vi "myRIO v1.0 Config Manager Encoder.vi"(7 "Action":T1, 10 "Encoder Signal Mode":T2, 11 "Encoder Channel":T3) -> (3 "Success?":bool)   [LabVIEW 2021]
uses:
  <vilib>/myRIO/Common/Instrument Driver Framework/myRIO v1.0/Encoder/typedefs/Encoder Channels Enum.ctl
  <vilib>/myRIO/Common/Instrument Driver Framework/myRIO v1.0/Encoder/typedefs/Encoder Signal Mode.ctl
  <vilib>/myRIO/Common/Instrument Driver Framework/myRIO v1.0/Encoder/typedefs/Encoder Config Manager Action Enum.ctl
  <vilib>/myRIO/Common/Instrument Driver Framework/myRIO v1.0/Encoder/typedefs/Encoder Config Cache Data.ctl
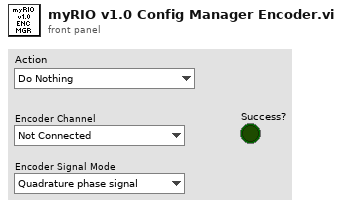
[diagram p1: front panel]
types:
  T1 = typedef "Encoder Config Manager Action Enum.ctl" = enum16{"Do Nothing", "Store", "Clear"}
  T2 = typedef "Encoder Signal Mode.ctl" = enum16{"Quadrature phase signal", "Step and direction signal"}
  T3 = typedef "Encoder Channels Enum.ctl" = enum16{"Not Connected", "C/ENC0", "C/ENC1", "A/ENC", "A/ENC0", "A/ENC1", "A/ENC2", "A/ENC3", "A/ENC4", "A/ENC5", "A/ENC6", "A/ENC7", "A/ENC8", "A/ENC9", "B/ENC", "B/ENC0", "B/ENC1", "B/ENC2", "B/ENC3", "B/ENC4", "B/ENC5", "B/ENC6", "B/ENC7", "B/ENC8", "B/ENC9", "DIO/ENC0", "DIO/ENC1", "DIO/ENC2", "DIO/ENC3", "DIO/ENC4"}
  T4 = typedef "Encoder Config Cache Data.ctl" = cluster{"Set?":bool, "Encoder Signal Mode":T2}
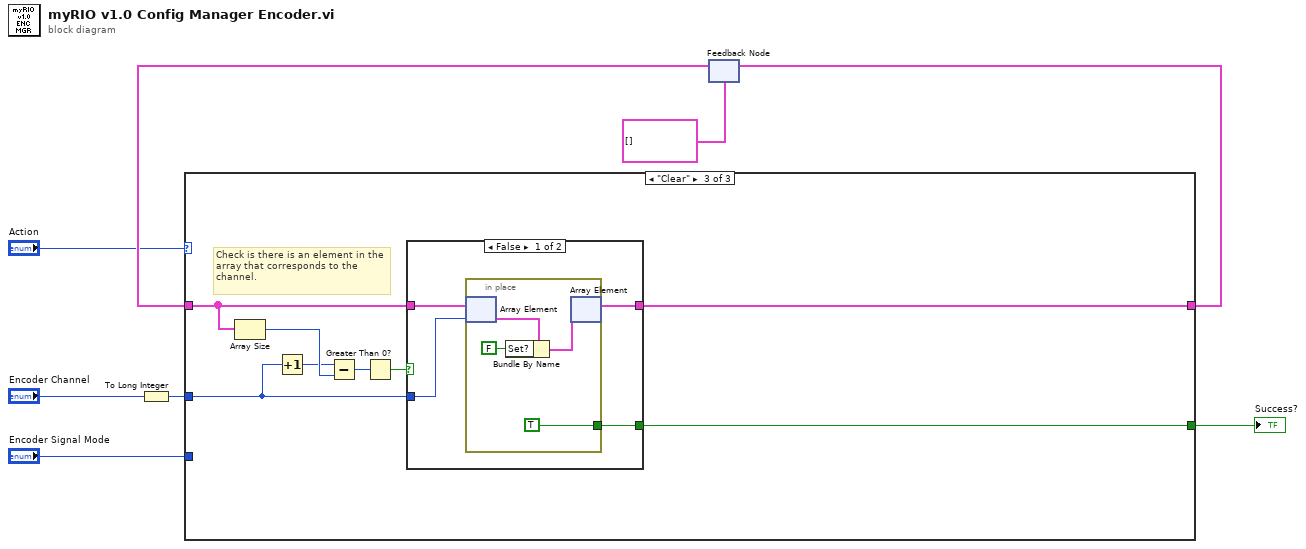
[diagram p0: block diagram]
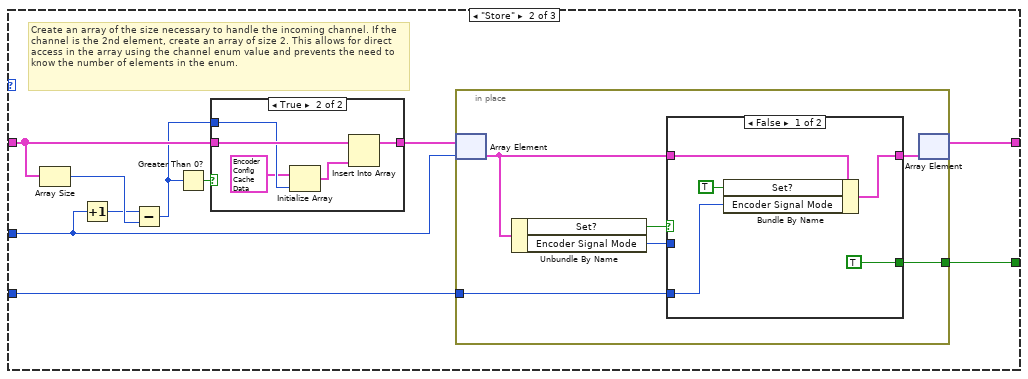
[diagram p3: hidden frame]
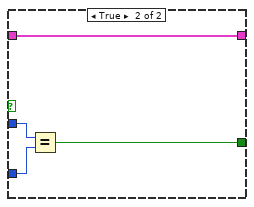
[diagram p5: hidden frame]
diagram:
  n1 = To Long Integer(number="Encoder Channel") -> (32bit integer=w3:i32)
  n2 = feedback #1(T4[] []) -> (w7:T4[])
  n3 = case shown="\"Clear\"" "Action" {
    tunnel: w7 -> [w9 w16 w45]
    tunnel: w3 -> [_ w11 w42]
    tunnel: "Encoder Signal Mode" -> [_ w19 _]
    tunnel: [w9 w18 w44] -> w5
    tunnel: [_ w10 w41] -> w2
    frame "Do Nothing", Default {
    }
    frame "Store" {
      # "Create an array of the size necessary to handle the incoming channel. If the channel is the 2nd element, create an array of size 2. This allows for direct access in the array using the channel enum value and prevents the need to know the number of elements in the enum."
      n4 = Array Size(array=w16) -> (size(s)=w15:i32)
      n5 = Increment(x=w11) -> (x+1=w12:i32)
      n6 = Subtract(x=w12, y=w15) -> (x-y=w14:i32)
      n7 = Greater Than 0?(x=w14) -> (x > 0?=w13:bool)
      n8 = case shown="True" w13 {
        tunnel: [w20 w24] -> w17
        tunnel: w16 -> [w20 w25]
        tunnel: w14 -> [_ w23]
        frame False {
        }
        frame True {
          n9 = Initialize Array(T4 {"Set?"=FALSE, "Encoder Signal Mode"=enum."Quadrature phase signal"}, w23) -> (w22:T4[])
          n10 = Insert Into Array(array=w25, new element=w22) -> (w24:T4[])  [unwired: 1 in]
        }
      }
      n11 = in-place {
        in-place-border: w19 -> [w29]
        in-place-border: [w26] -> w10
        n12 = in-place-array #2(w17, w11) -> (w28:T4)
        n13 = Unbundle By Name(w28) -> ("Set?"=w31:bool, "Encoder Signal Mode"=w30:T2)
        n14 = case shown="False" w31 {
          tunnel: w30 -> [_ w40]
          tunnel: w29 -> [w34 w39]
          tunnel: w28 -> [w36 w38]
          tunnel: [w35 w38] -> w27
          tunnel: [TRUE ("Set?") w37] -> w26
          frame False {
            n15 = Bundle By Name(cluster=w36, "Set?"=TRUE, "Encoder Signal Mode"=w34) -> (w35:T4)
          }
          frame True {
            n16 = Equal?(x=w40, y=w39) -> (x = y?=w37:bool)
          }
        }
        n17 = in-place-array #2(w27) -> (w18:T4[])  [unwired: 1 out]
      }
    }
    frame "Clear" {
      # "Check is there is an element in the array that corresponds to the channel."
      n18 = Array Size(array=w45) -> (size(s)=w48:i32)
      n19 = Increment(x=w42) -> (x+1=w46:i32)
      n20 = Subtract(x=w46, y=w48) -> (x-y=w47:i32)
      n21 = Greater Than 0?(x=w47) -> (x > 0?=w43:bool)
      n22 = case shown="False" w43 {
        tunnel: [w51 w57] -> w44
        tunnel: w45 -> [w52 w57]
        tunnel: w42 -> [w50 _]
        tunnel: [w49 _] -> w41
        frame False {
          n23 = in-place {
            in-place-border: [TRUE ("Set?")] -> w49
            n24 = in-place-array #3(w52, w50) -> (w56:T4)
            n25 = Bundle By Name(cluster=w56, "Set?"=FALSE) -> (w55:T4)
            n26 = in-place-array #3(w55) -> (w51:T4[])  [unwired: 1 out]
          }
        }
        frame True {
          # "If there is no element in the array for the channel then it cannot be cleared so the Clear operation is unsuccessful."
        }
      }
    }
  }
  "Success?" <- w2
  n27 = feedback-in #1(w5) -> ()
